vi "Resizing.vi"() -> ()   [LabVIEW 2011]
uses:
  <vilib>/Heliosphere Research LLC/Advanced Plotting Toolkit/Advanced Plotting Toolkit.lvlib
  <vilib>/Heliosphere Research LLC/Advanced Plotting Toolkit/typedefs/PlotColor.ctl
  <vilib>/Heliosphere Research LLC/Advanced Plotting Toolkit/properties/Line_Style.ctl
  <vilib>/Heliosphere Research LLC/Advanced Plotting Toolkit/properties/Line.ctl
  <vilib>/Heliosphere Research LLC/Advanced Plotting Toolkit/properties/Display.ctl
  <vilib>/Heliosphere Research LLC/Advanced Plotting Toolkit/api_plotting/BarProperties.ctl
  <vilib>/Heliosphere Research LLC/Advanced Plotting Toolkit/api_core/NewPlotProperties.ctl
panel:
  in  "DPI":dbl=80.0
  in  "Height (pixels)":dbl=240.0
  in  "Width (pixels)":dbl=320.0
  in  "Fit to Picture":bool
  out "Bar Plot":picture
  # "Resizing"
  # "Every plot in the Toolkit has a width and height in pixels, which\ndefaults to 640 x 480.  Because many items like fonts, line\nthicknesses, marker sizes, etc., have widths in \"points\" (1/72\ninch), every plot also has an associated DPI or \"dots-per-inch\"\nvalue which translates inch-based measurements to pixels.\n\nWhen saving to an \"inch-based\" format like PDF, the DPI value\nis also used to translate pixel-based quantities (like the plot\nwidth and height) to inches.\n\nSize.vi allows you to change the plot width, height, or DPI.  In\nthis example, the plot is created with a dark background, to make\nthe edge of the plot clearly visible.  Try changing the size and\nDPI values below.  There's also an auto-sizing feature on\nView.vi, to exactly resize the plot for an existing Picture control.\n\nThanks to the Toolkit's use of vector art internally, plots can be\narbitrarily and repeatedly resized without loss of detail."
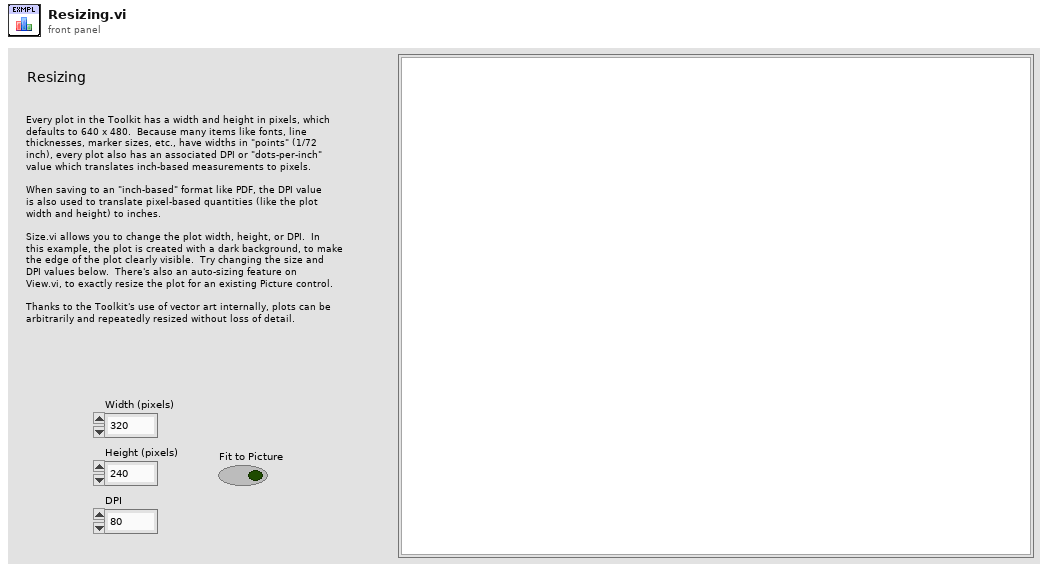
[diagram p1: front panel]
types:
  T1 = typedef "Advanced Plotting Toolkit.lvlib/NewPlotProperties.ctl" = cluster{"Background Color":T2, "Axis Background":T2, "Left Margin":dbl, "Right Margin":dbl, "Bottom Margin":dbl, "Top Margin":dbl, "Aspect Ratio":dbl}
  T2 = typedef "Advanced Plotting Toolkit.lvlib/PlotColor.ctl" = u32
  T3 = typedef "Advanced Plotting Toolkit.lvlib/BarProperties.ctl" = cluster{"Bar Color":T2, "Line":T4, "Display":T6}
  T4 = typedef "Advanced Plotting Toolkit.lvlib/Line.ctl" = cluster{"Style":T5, "Color":T2, "Width":sgl}
  T5 = typedef "Advanced Plotting Toolkit.lvlib/Line_Style.ctl" = enum16{"Automatic", "Solid", "Dashed", "Dotted", "Dash-dot", "Invisible"}
  T6 = typedef "Advanced Plotting Toolkit.lvlib/Display.ctl" = cluster{"Alpha":dbl, "Z Order":dbl}
  T7 = typedef "Advanced Plotting Toolkit.lvlib/PlotID.ctl" = i32
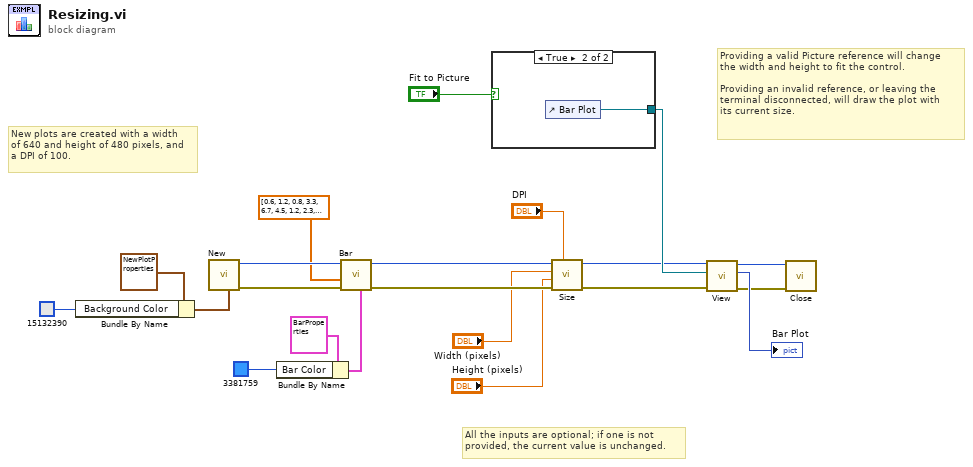
[diagram p0: block diagram]
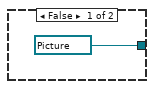
[diagram p2: hidden frame]
diagram:
  # "All the inputs are optional; if one is not\nprovided, the current value is unchanged."
  # "New plots are created with a width\nof 640 and height of 480 pixels, and\na DPI of 100."
  # "Providing a valid Picture reference will change\nthe width and height to fit the control.\n\nProviding an invalid reference, or leaving the\nterminal disconnected, will draw the plot with\nits current size."
  n1 = Bundle By Name(cluster=T1 {"Background Color"=2147483647, "Axis Background"=2147483647, "Left Margin"=nan, "Right Margin"=nan, "Bottom Margin"=nan, "Top Margin"=nan, "Aspect Ratio"=nan} ("New Plot Properties"), "Background Color"=u32 15132390 ("Bar Color")) -> (w11:T1)
  n2 = call <vilib>:"New.vi"("Properties"=w11) -> ("error out"=w19:errorcluster, "Plot ID"=w20:T7)  [unwired: 9 in]
  n3 = Bundle By Name(cluster=T3 {"Bar Color"=2147483647, "Line"={"Style"=enum."Automatic", "Color"=2147483647, "Width"=nan}, "Display"={"Alpha"=nan, "Z Order"=nan}} ("Bar Plot Properties"), "Bar Color"=u32 3381759) -> (w16:T3)
  n4 = call <vilib>:"Bar.vi"("Properties"=w16, "error in (no error)"=w19, "Bar Lengths"=dbl[] [0.6, 1.2, 0.8, 3.3, 6.7, 4.5, 1.2, 2.3, 4.4, 1.9, 2.1, 2.3, 3.4, 1.2, 1.1] ("Bar Data"), "Plot ID"=w20) -> ("error out"=w7:errorcluster, "Plot ID Out"=w8:T7)  [unwired: 6 in]
  n5 = case shown="True" "Fit to Picture" {
    tunnel: [refnum<vi> refnum ("Bar Plot 2") w23] -> w9
    frame False {
    }
    frame True {
      n6 = control-ref of="Bar Plot"() -> (w23:refnum<vi>)
    }
  }
  n7 = call <vilib>:"Size.vi"("DPI"="DPI", "error in (no error)"=w7, "Height (pixels)"="Height (pixels)", "Width (pixels)"="Width (pixels)", "Plot ID"=w8) -> ("error out"=w5:errorcluster, "Plot ID Out"=w6:T7)  [unwired: 5 in]
  n8 = call <vilib>:"View.vi"("error in (no error)"=w5, "Ref for Sizing"=w9, "Plot ID"=w6) -> ("error out"=w1:errorcluster, "Picture"=→"Bar Plot":picture, "Plot ID Out"=w18:T7)  [unwired: 6 in]
  n9 = call <vilib>:"Close.vi"("error in (no error)"=w1, "Plot ID"=w18) -> ()  [unwired: 9 in, 1 out]
